vi "CreateIntegerArray.vi"(10 "Input Values":T1) -> (2 "Output Array":i32[](array[numeric]))   [LabVIEW 2014]
uses:
  <vilib>/imath/engines/lvmath2/RunTimeEngine/Managers/WorkSpace/UID Generator.vi
  <vilib>/imath/engines/lvmath2/RunTimeSupport/NIMS_Complex To Real.vi
  <instcachedir>/0/NIMS_Complex To Real_CFEFC05793354143908F7AF8F5FCAA9D.lvgen/NIMS_Complex To Real_CFEFC05793354143908F7AF8F5FCAA9D_001.vi
  <vilib>/imath/engines/lvmath2/RunTimeEngine/BuiltInFunctions/logramp/NIMS_logramp.vi
  <vilib>/imath/engines/lvmath2/RunTimeEngine/RunTimeType/NIMS_RunTimeType_From StrictType (excl LVString).vi
  <instcachedir>/0/NIMS_RunTimeType_From StrictType (excl LVString)_15A5391EEA9C4AACB9955AC755B83D29.lvgen/NIMS_RunTimeType_From StrictType (excl LVString)_15A5391EEA9C4AACB9955AC755B83D29_000.vi
  <vilib>/imath/engines/lvmath2/RunTimeEngine/ErrorHandling/NIMS_Create Error From Enums.vi
  <vilib>/imath/engines/lvmath2/RunTimeEngine/LocalVariableDefStatement/MC_LocalVariableDefStatement_Display.vi
  <vilib>/imath/engines/lvmath2/RunTimeEngine/BuiltInFunctions/linramp/NIMS_linramp.vi
  <vilib>/imath/engines/lvmath2/RunTimeEngine/Managers/SymbolTable/Clear UID.vi
  <vilib>/imath/engines/lvmath2/RunTimeEngine/NodeEndStatement/NIMS_NodeEndStatement_Output.vi
  <instcachedir>/0/NIMS_NodeEndStatement_Output_53EC0D466D134D7ABD903AC30B43404B.lvgen/NIMS_NodeEndStatement_Output_53EC0D466D134D7ABD903AC30B43404B_005.vi
  <vilib>/imath/engines/lvmath2/RunTimeEngine/ErrorHandling/NIMS_Finalize Error.vi
  <vilib>/imath/engines/lvmath2/RunTimeEngine/Managers/SymbolTable/NIMS_WorkSpace.lvlib
panel:
  # "Takes in a max, min, # of points, and type of spacing and outputs an integer array"
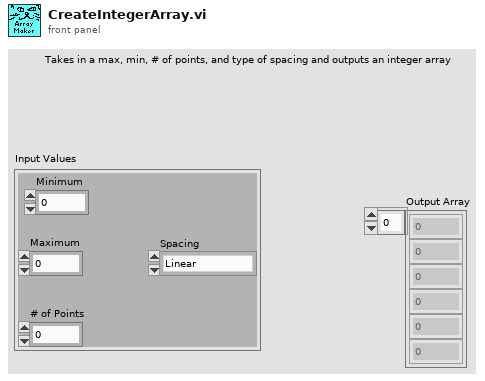
[diagram p1: front panel]
types:
  T1 = cluster{"Minimum":i32, "Maximum":i32, "# of Points":i32, "Spacing":enum16{"Linear", "Logarithmic"}}
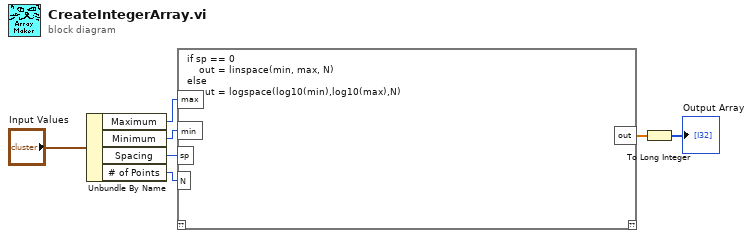
[diagram p0: block diagram]
diagram:
  n1 = Unbundle By Name("Input Values") -> ("Maximum"=w4:i32, "Minimum"=w3:i32, "Spacing"=w2:enum16{"Linear", "Logarithmic"}, "# of Points"=w1:i32)
  n2 = mathscript code="if sp == 0\n    out = linspace(min, max, N)\nelse\n    out = logspace(log10(min),log10(max),N)\nend"("max"=w4, "min"=w3, "sp"=w2, "N"=w1) -> ("out"=w7:dbl[])  [unwired: 1 in, 1 out]
  n3 = To Long Integer(number=w7) -> (32bit integer=→"Output Array":i32[])
